vi "Keypad backlight.vi"(8 "error in (no error)":errorcluster, 10 "BKLT":u32(ring) items=["Off", "Low", "High"], 11 "VISA resource name":refnum<visa-resource-name>) -> (0 "error out":errorcluster, 3 "VISA resource name out":refnum<visa-resource-name>)   [LabVIEW 2012, in "Newport 1830-C.lvlib"]
doc: "0=Off\n1=Low\n2=high"
uses:
  Newport 1830-C.lvlib
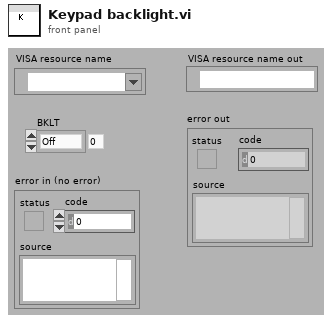
[diagram p1: front panel]
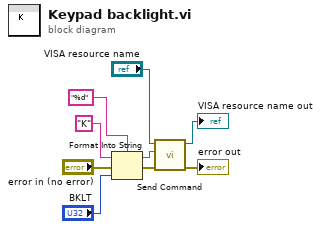
[diagram p0: block diagram]
diagram:
  n1 = Format Into String(format string="%d", initial string="K" ("command"), error in="error in (no error)", "BKLT") -> (resulting string=w5:string, error out=w6:errorcluster)
  n2 = call "Send Command.vi"("error in (no error)"=w6, "write buffer"=w5, "VISA resource name In"="VISA resource name") -> ("error out"=→"error out":errorcluster, "VISA resource name out"=→"VISA resource name out":refnum<visa-resource-name>)  [unwired: 7 in]
